vi "EventListener.vi"(9 "Amount":string, 10 "Account No.":string, 11 "Cases":string) -> ()   [LabVIEW 2023]
panel:
  out "Event":string
  out "current time":timestamp
  in  "error in":errorcluster
  out "error out":errorcluster
  # "Auto-generated Content"
  # "Errors"
  # "Input"
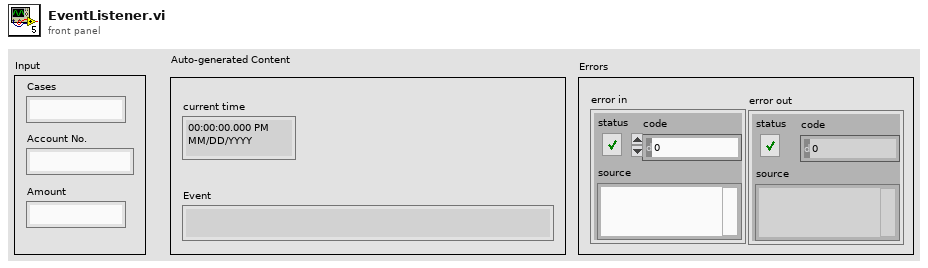
[diagram p1: front panel]
types:
  T1 = enum16{"open", "replace", "create", "open or create", "replace or create", "replace or create with confirmation"}
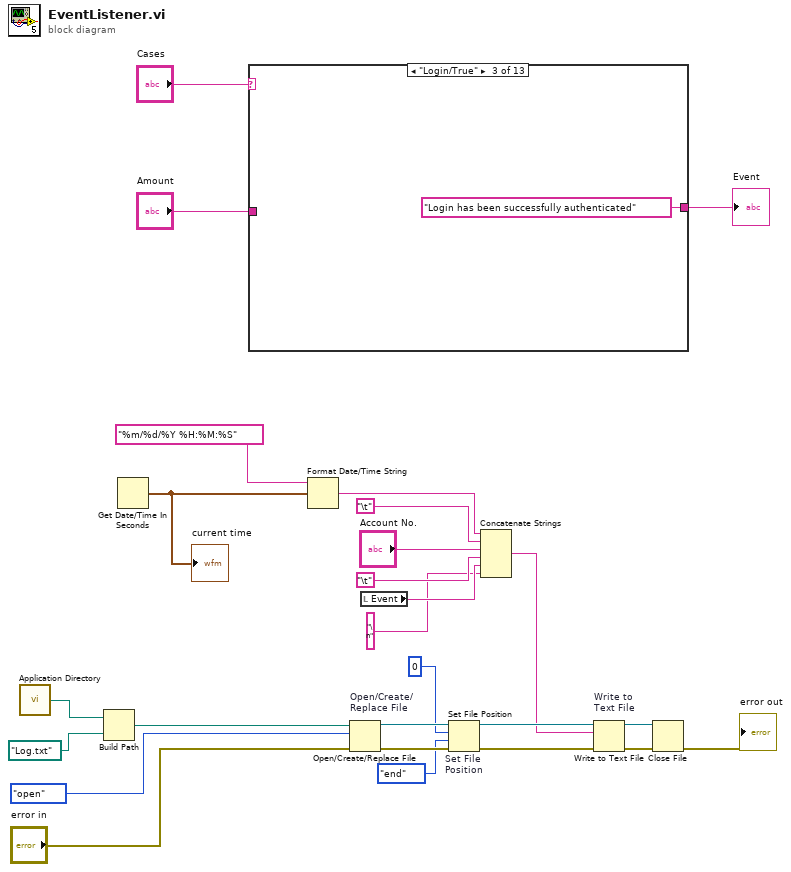
[diagram p0: block diagram]
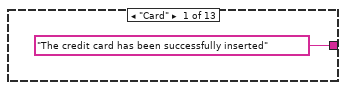
[diagram p2: hidden frame]
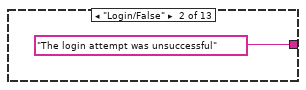
[diagram p3: hidden frame]
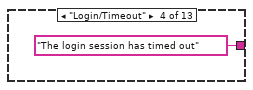
[diagram p4: hidden frame]
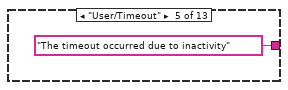
[diagram p5: hidden frame]
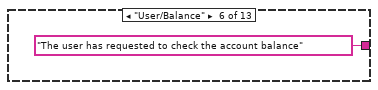
[diagram p6: hidden frame]
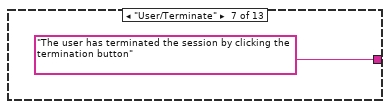
[diagram p7: hidden frame]
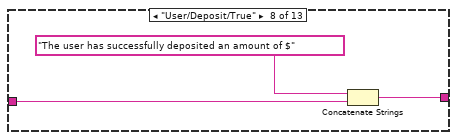
[diagram p8: hidden frame]
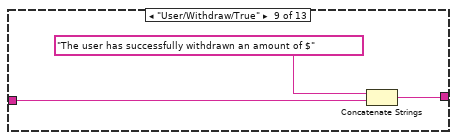
[diagram p9: hidden frame]
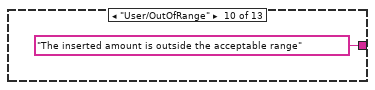
[diagram p10: hidden frame]
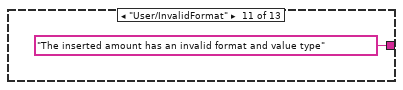
[diagram p11: hidden frame]
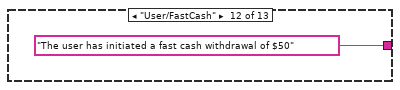
[diagram p12: hidden frame]
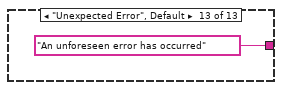
[diagram p13: hidden frame]
diagram:
  n1 = call <vilib>:"Application Directory.vi"() -> ("Application Directory"=w26:path)
  n2 = Build Path(base path=w26, name or relative path=path "Log.txt") -> (appended path=w14:path)
  n3 = Get Date/Time In Seconds() -> (seconds since 1Jan1904=w24:timestamp)
  "current time" <- w24
  n4 = case shown="\"Login/True\"" "Cases" {
    tunnel: "Amount" -> [_ _ _ _ _ _ _ w35 w38 _ _ _ _]
    tunnel: ["The credit card has been successfully inserted" "The login attempt was unsuccessful" "Login has been successfully authenticated" "The login session has timed out" "The timeout occurred due to inactivity" "The user has requested to check the account balance" "The user has terminated the session by clicking the termination button" w34 w37 "The inserted amount is outside the acceptable range" "The inserted amount has an invalid format and value type" "The user has initiated a fast cash withdrawal of $50" "An unforeseen error has occurred"] -> w20
    frame "Card" {
    }
    frame "Login/False" {
    }
    frame "Login/True" {
    }
    frame "Login/Timeout" {
    }
    frame "User/Timeout" {
    }
    frame "User/Balance" {
    }
    frame "User/Terminate" {
    }
    frame "User/Deposit/True" {
      n5 = Concatenate Strings("The user has successfully deposited an amount of $" ("string"), w35) -> (w34:string)
    }
    frame "User/Withdraw/True" {
      n6 = Concatenate Strings("The user has successfully withdrawn an amount of $" ("string"), w38) -> (w37:string)
    }
    frame "User/OutOfRange" {
    }
    frame "User/InvalidFormat" {
    }
    frame "User/FastCash" {
    }
    frame "Unexpected Error", Default {
    }
  }
  "Event" <- w20
  n7 = Format Date/Time String(time format string (%c)="%m/%d/%Y %H:%M:%S", seconds (now)=w24) -> (date/time string=w19:string)  [unwired: 1 in]
  n8 = Open/Create/Replace File "Open/Create/\nReplace File"(file path (use dialog)=w14, error in="error in", operation (0:open)=T1."open") -> (refnum out=w8:refnum<file>, error out=w7:errorcluster)  [unwired: 3 in, 1 out]
  n9 = local read "Event"() -> (w15:string)
  n10 = Set File Position "Set File \nPosition"(offset (in bytes) (0)=i64 0, refnum=w8, from (0:start)=enum16{"start", "end", "current"}."end", error in=w7) -> (refnum out=w4:refnum<file>, error out=w3:errorcluster)
  n11 = Concatenate Strings(w19, "\t", "Account No.", "\t", w15, "\n" ("string")) -> (w2:string)
  n12 = Write to Text File "Write to \nText File"(file (use dialog)=w4, text=w2, error in=w3) -> (refnum out=w12:refnum<file>, error out=w13:errorcluster)  [unwired: 1 in, 1 out]
  n13 = Close File(refnum=w12, error in=w13) -> (error out=→"error out":errorcluster)  [unwired: 1 out]
